vi "DataToChaine.vi"(11 "X":string) -> (3 "\"X\"":string)   [LabVIEW 2020]
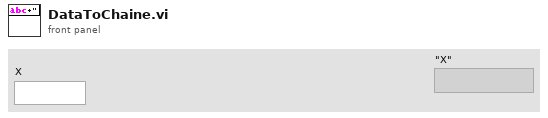
[diagram p1: front panel]
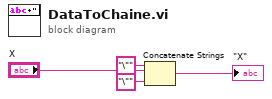
[diagram p0: block diagram]
diagram:
  n1 = Concatenate Strings("\"" ("chaîne"), "X", "\"" ("chaîne")) -> (→"\"X\"":string)
